vi "Demo.vi"   [LabVIEW 2021]
uses:
  Z:/Samples Yaskawa/LabVIEW/Library/UnderAutomation.Yaskawa.dll
  Library/UnderAutomation.Yaskawa.dll
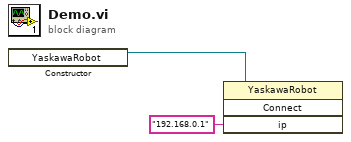
[diagram p0: block diagram]
diagram:
  n1 = constructor class="YaskawaRobot"() -> (reference out=w2:refnum<k24>)  [unwired: 3 in, 2 out]
  n2 = invoke class="YaskawaRobot" method="Connect"(reference=w2, "ip"="192.168.0.1") -> ()  [unwired: 2 in, 4 out]
